vi "KB-WriteTitle.vi"() -> ()   [LabVIEW 2015]
uses:
  <vilib>/Utility/file.llb/Write Delimited Spreadsheet (string).vi
  <vilib>/Utility/file.llb/Read Delimited Spreadsheet (string).vi
panel:
  out "数组 6":string[](array[string])
  out "数组 5":string[](array[string])
  out "已删除的部分":string[](array[string])
  out "数组 4":string[][](array[string])
  out "x*y":dbl
  out "数组 3":string[][](array[string])
  out "x/y":dbl
  out "大小":i32
  out "数组 2":string[](array[string])
  out "数组":string[](array[string])
  in  "子数组":string[](array[string])=["ITEM-(Offset)O-I", "ITEM-(Offset)I", "ITEM-(Offset)O", "ITEM-同心度", "ITEM-颜色", "ITEM-是否漏装", "ITEM-(Offset)O-I", "ITEM-(Offset)I", "ITEM-(Offset)O", "ITEM-同心度", "ITEM-颜色", "ITEM-是否漏装", "ITEM-(Offset)O-I", "ITEM-(Offset)I", "ITEM-(Offset)O", "ITEM-同心度", "ITEM-颜色", "ITEM-是否漏装", "ITEM-(Offset)O-I", "ITEM-(Offset)I", "ITEM-(Offset)O", "ITEM-同心度", "ITEM-颜色", "ITEM-是否漏装", "ITEM-(Offset)O-I", "ITEM-(Offset)I", "ITEM-(Offset)O", "ITEM-同心度", "ITEM-颜色", "ITEM-是否漏装", "ITEM-(Offset)O-I", "ITEM-(Offset)I", "ITEM-(Offset)O", "ITEM-同心度", "ITEM-颜色", "ITEM-是否漏装", "ITEM-(Offset)O-I", "ITEM-(Offset)I", "ITEM-(Offset)O", "ITEM-同心度", "ITEM-颜色", "ITEM-是否漏装", "ITEM-(Offset)O-I", "ITEM-(Offset)I", "ITEM-(Offset)O", "ITEM-同心度", "ITEM-颜色", "ITEM-是否漏装", "ITEM-(Offset)O-I", "ITEM-(Offset)I", "ITEM-(Offset)O", "ITEM-同心度", "ITEM-颜色", "ITEM-是否漏装", "ITEM-(Offset)O-I", "ITEM-(Offset)I", "ITEM-(Offset)O", "ITEM-同心度", "ITEM-颜色", "ITEM-是否漏装", "ITEM-(Offset)O-I", "ITEM-(Offset)I", "ITEM-(Offset)O", "ITEM-同心度", "ITEM-颜色", "ITEM-是否漏装", "ITEM-(Offset)O-I", "ITEM-(Offset)I", "ITEM-(Offset)O", "ITEM-同心度", "ITEM-颜色", "ITEM-是否漏装", "ITEM-(Offset)O-I", "ITEM-(Offset)I", "ITEM-(Offset)O", "ITEM-同心度", "ITEM-颜色", "ITEM-是否漏装", "ITEM-(Offset)O-I", "ITEM-(Offset)I", "ITEM-(Offset)O", "ITEM-同心度", "ITEM-颜色", "ITEM-是否漏装", "ITEM-(Offset)O-I", "ITEM-(Offset)I", "ITEM-(Offset)O", "ITEM-同心度", "ITEM-颜色", "ITEM-是否漏装", "ITEM-(Offset)O-I", "ITEM-(Offset)I", "ITEM-(Offset)O", "ITEM-同心度", "ITEM-颜色", "ITEM-是否漏装", "ITEM-(Offset)O-I", "ITEM-(Offset)I", "ITEM-(Offset)O", "ITEM-同心度", "ITEM-颜色", "ITEM-是否漏装", "ITEM-(Offset)O-I", "ITEM-(Offset)I", "ITEM-(Offset)O", "ITEM-同心度", "ITEM-颜色", "ITEM-是否漏装", "ITEM-(Offset)O-I", "ITEM-(Offset)I", "ITEM-(Offset)O", "ITEM-同心度", "ITEM-颜色", "ITEM-是否漏装", "ITEM-(Offset)O-I", "ITEM-(Offset)I", "ITEM-(Offset)O", "ITEM-同心度", "ITEM-颜色", "ITEM-是否漏装", "ITEM-(Offset)O-I", "ITEM-(Offset)I", "ITEM-(Offset)O", "ITEM-同心度", "ITEM-颜色", "ITEM-是否漏装", "ITEM-(Offset)O-I", "ITEM-(Offset)I", "ITEM-(Offset)O", "ITEM-同心度", "ITEM-颜色", "ITEM-是否漏装", "ITEM-(Offset)O-I", "ITEM-(Offset)I", "ITEM-(Offset)O", "ITEM-同心度", "ITEM-颜色", "ITEM-是否漏装", "ITEM-(Offset)O-I", "ITEM-(Offset)I", "ITEM-(Offset)O", "ITEM-同心度", "ITEM-颜色", "ITEM-是否漏装", "ITEM-(Offset)O-I", "ITEM-(Offset)I", "ITEM-(Offset)O", "ITEM-同心度", "ITEM-颜色", "ITEM-是否漏装", "ITEM-(Offset)O-I", "ITEM-(Offset)I", "ITEM-(Offset)O", "ITEM-同心度", "ITEM-颜色", "ITEM-是否漏装", "ITEM-(Offset)O-I", "ITEM-(Offset)I", "ITEM-(Offset)O", "ITEM-同心度", "ITEM-颜色", "ITEM-是否漏装", "ITEM-(Offset)O-I", "ITEM-(Offset)I", "ITEM-(Offset)O", "ITEM-同心度", "ITEM-颜色", "ITEM-是否漏装", "ITEM-(Offset)O-I", "ITEM-(Offset)I", "ITEM-(Offset)O", "ITEM-同心度", "ITEM-颜色", "ITEM-是否漏装", "ITEM-(Offset)O-I", "ITEM-(Offset)I", "ITEM-(Offset)O", "ITEM-同心度", "ITEM-颜色", "ITEM-是否漏装", "ITEM-(Offset)O-I", "ITEM-(Offset)I", "ITEM-(Offset)O", "ITEM-同心度", "ITEM-颜色", "ITEM-是否漏装"]
  out "all rows":string[][](array[string]) caption="所有行"
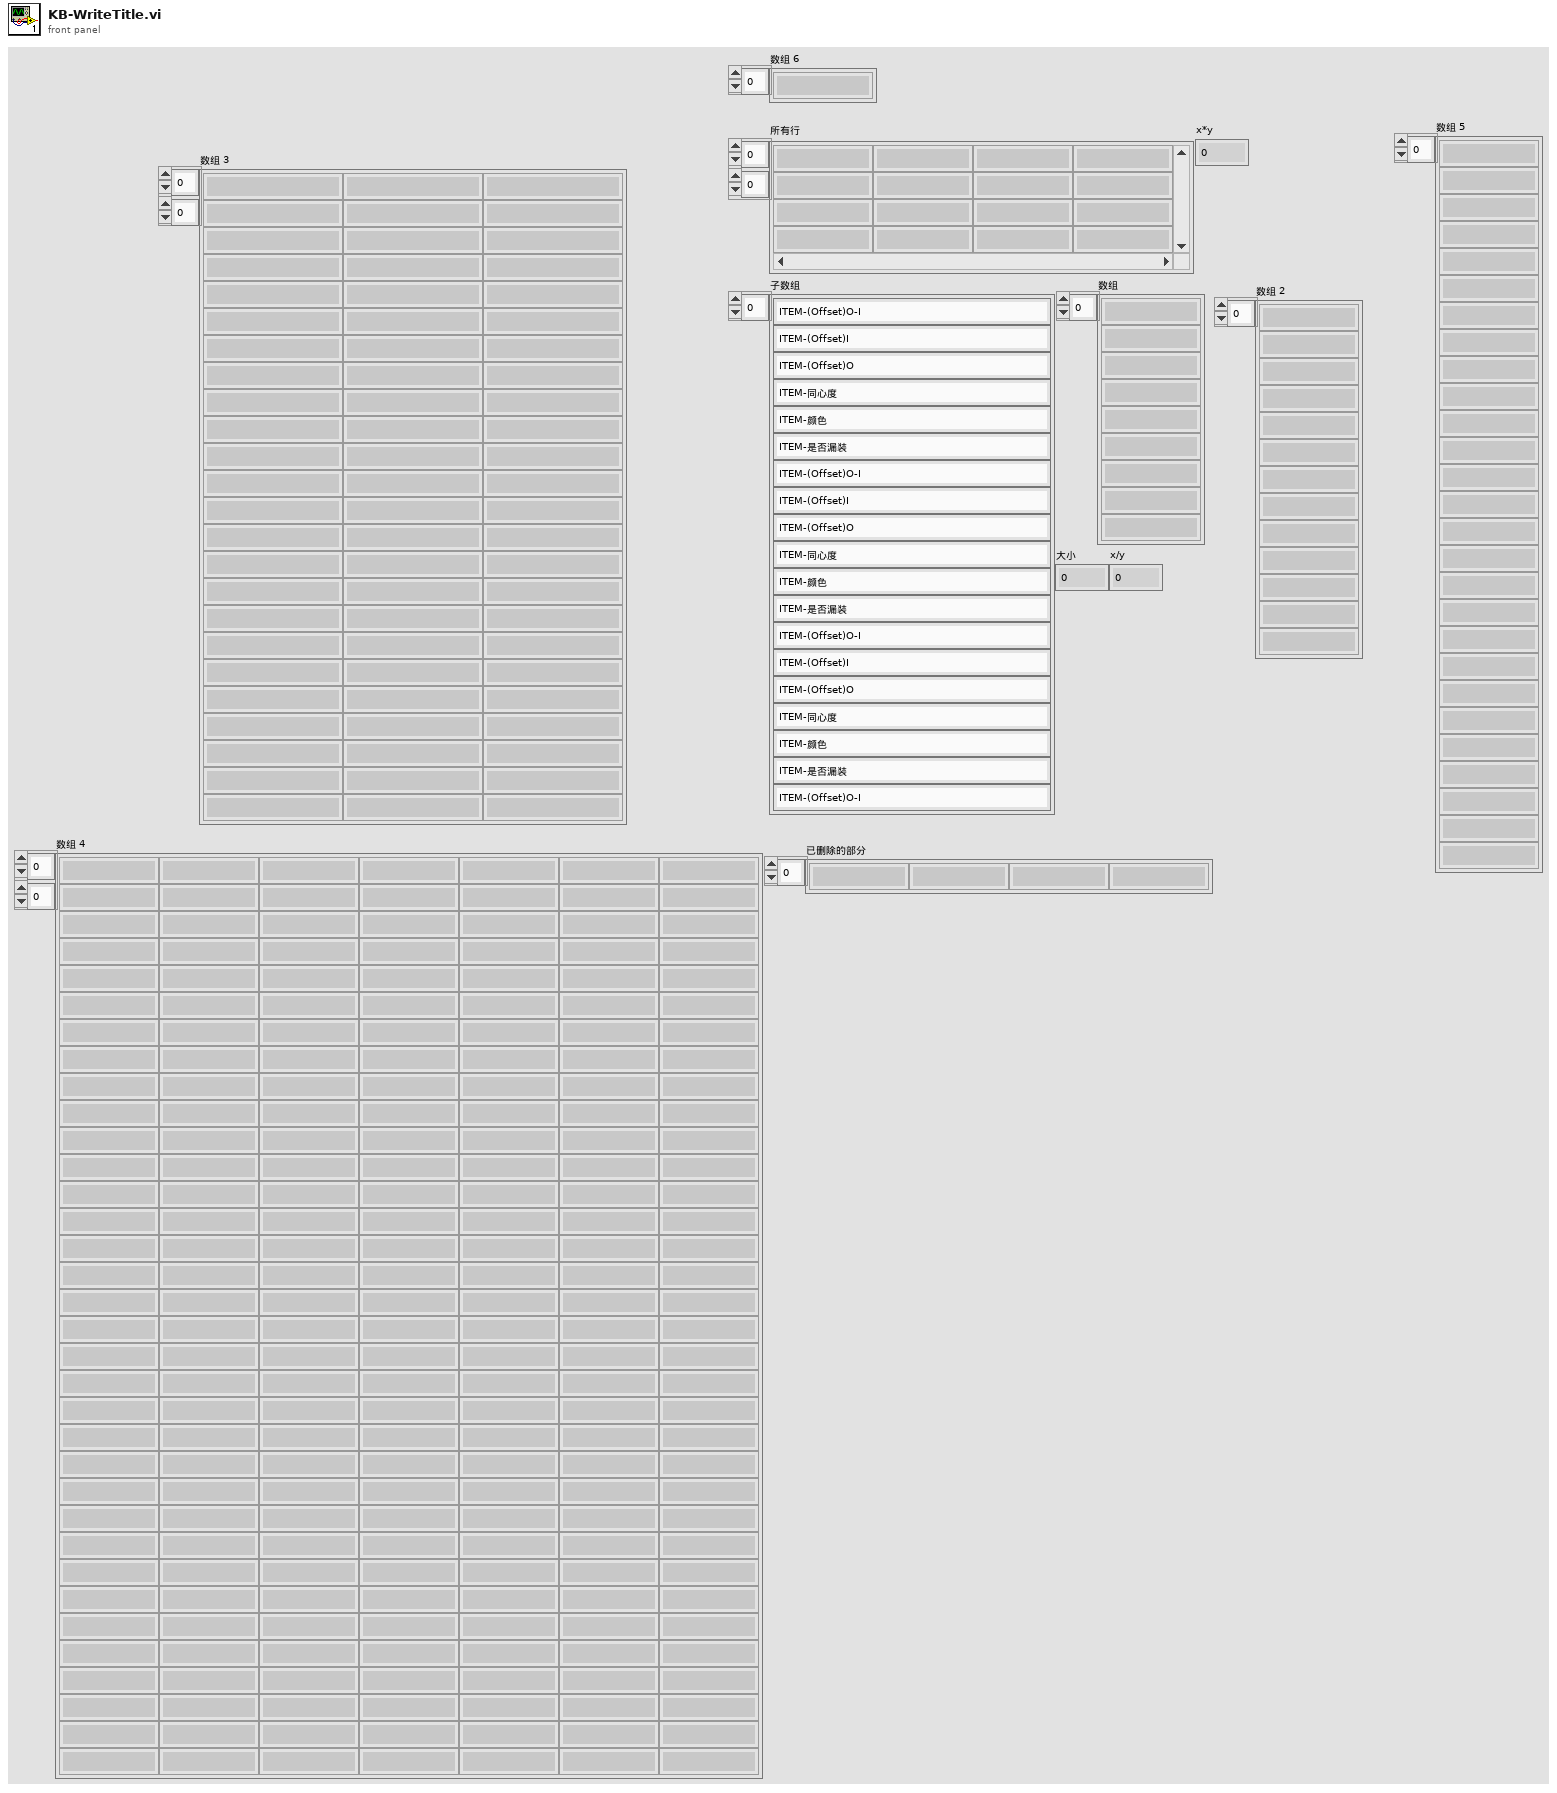
[diagram p1: front panel]
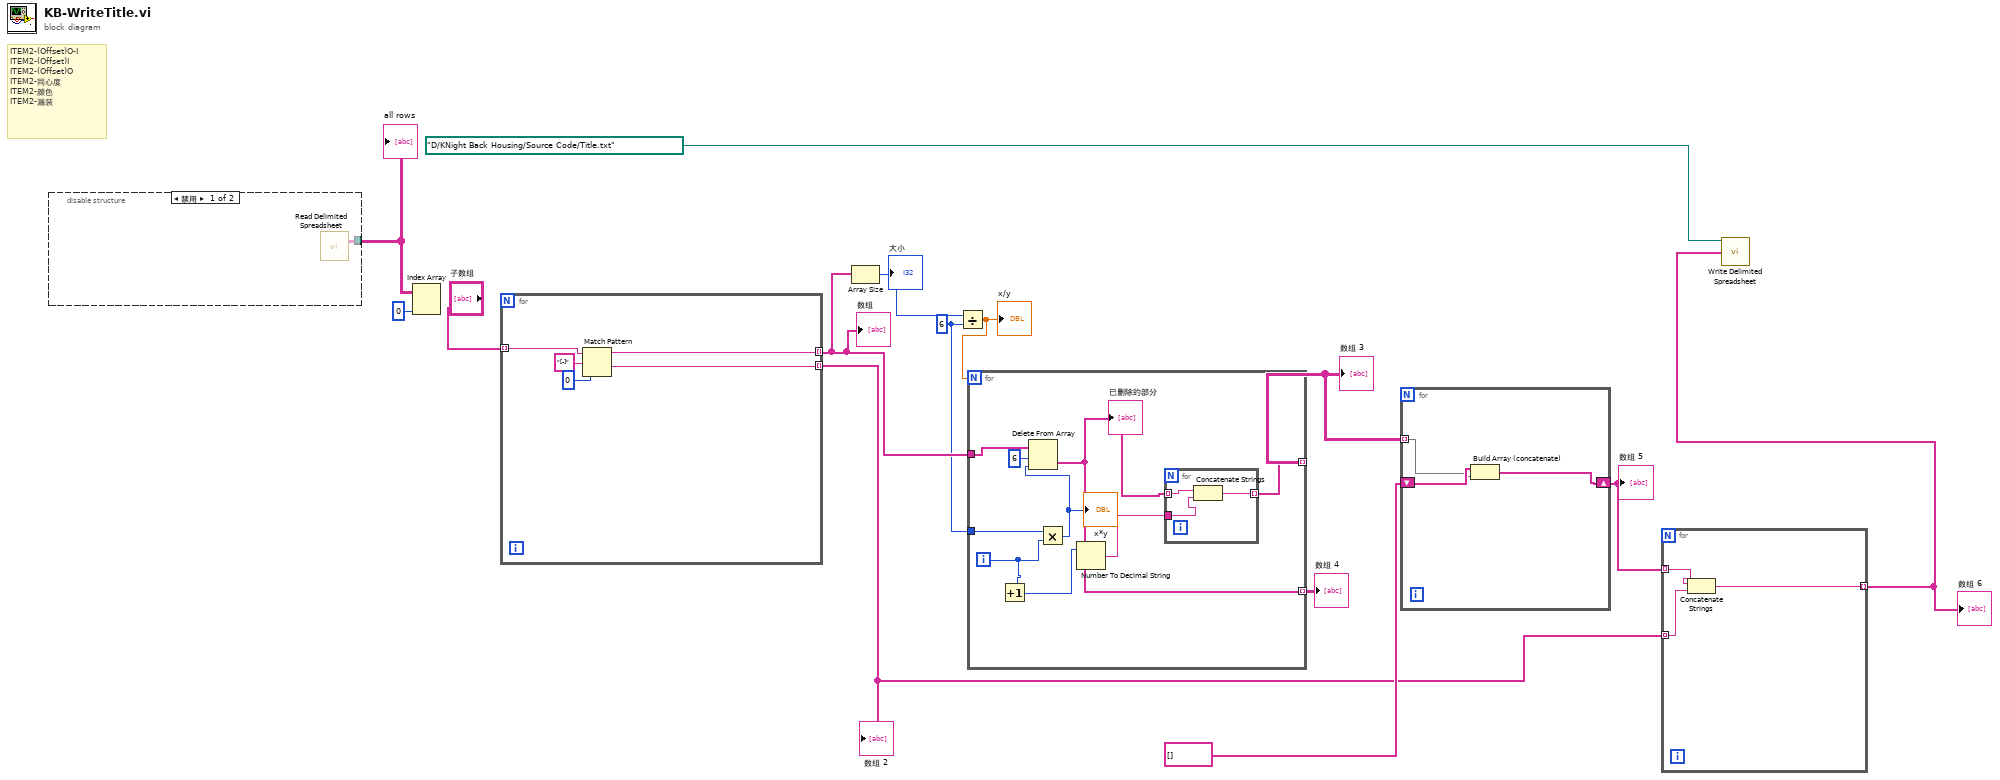
[diagram p0: block diagram]
diagram:
  w8 = 6 ("y")
  # "ITEM2-(Offset)O-I\nITEM2-(Offset)I\nITEM2-(Offset)O\nITEM2-同心度\nITEM2-颜色\nITEM2-漏装"
  n1 = disable-structure shown="禁用" {
    disable-tunnel: [w16 _] -> w14
    disable-tunnel: _ -> [w15 _]
    frame Disabled {
      n2 = call-poly <vilib>:"Read Delimited Spreadsheet.vi"("file path (dialog if empty)"=w15) -> ("all rows"=w16:string[][])  [unwired: 9 in, 5 out]
    }
    frame Enabled {
    }
  }
  "all rows" <- w14
  n3 = Index Array(array=w14, index (col)=0 ("禁用的索引 (列)")) -> ()  [unwired: 1 in, 1 out]
  n4 = for {
    tunnel: "子数组" -> [w21] mode=indexing
    tunnel: [w18] -> w9 mode=indexing
    tunnel: [w17] -> w2 mode=indexing
    n5 = Match Pattern(string=w21, regular expression="[-]" ("正则表达式"), offset (0)=0 ("偏移量(0)")) -> (before substring=w18:string, after substring=w17:string)  [unwired: 2 out]
  }
  "数组" <- w9
  "数组 2" <- w2
  n6 = Array Size(array=w9) -> (size(s)=w11:i32)
  "大小" <- w11
  n7 = Divide(x=w11, y=w8) -> (x/y=w10:dbl)
  "x/y" <- w10
  n8 = for {
    N: w10 -> [_]
    tunnel: w8 -> [w30]
    tunnel: w9 -> [w29]
    tunnel: [w25] -> w6 mode=indexing
    tunnel: [w24] -> w7 mode=indexing
    i -> [w23]
    n9 = Increment(x=w23) -> (x+1=w22:i32)
    n10 = Multiply(x=w30, y=w23) -> (x*y=w27:i32)
    "x*y" <- w27
    n11 = Delete From Array(array=w29, length=6 ("长度"), index=w27) -> (deleted portion=w24:string[])  [unwired: 1 out]
    "已删除的部分" <- w24
    n12 = Number To Decimal String(number=w22) -> (decimal integer string=w26:string)  [unwired: 1 in]
    n13 = for {
      tunnel: w24 -> [w33] mode=indexing
      tunnel: w26 -> [w32]
      tunnel: [w31] -> w25 mode=indexing
      n14 = Concatenate Strings(w33, w32) -> (w31:string)
    }
  }
  "数组 3" <- w6
  "数组 4" <- w7
  n15 = for {
    tunnel: w6 -> [w35] mode=indexing
    shift-right: [w34] -> w3
    shift-left: string[] [] -> [w36]
    n16 = Build Array (concatenate)(w36, w35) -> (w34:string[])
  }
  "数组 5" <- w3
  n17 = for {
    tunnel: w3 -> [w39] mode=indexing
    tunnel: w2 -> [w38] mode=indexing
    tunnel: [w37] -> w1 mode=indexing
    n18 = Concatenate Strings(w39, w38) -> (w37:string)
  }
  "数组 6" <- w1
  n19 = call-poly <vilib>:"Write Delimited Spreadsheet.vi"("file path (dialog if empty)"=path "D:/KNight Back Housing/Source Code/Title.txt", "1D data"=w1) -> ()  [unwired: 12 in, 2 out]
